vi "ArrayLast_D.vi"(11 "1D Array In":dbl[](array[numeric])) -> (0 "Last Element":dbl, 1 "Head of Array":dbl[](array[numeric]))   [LabVIEW 2009]
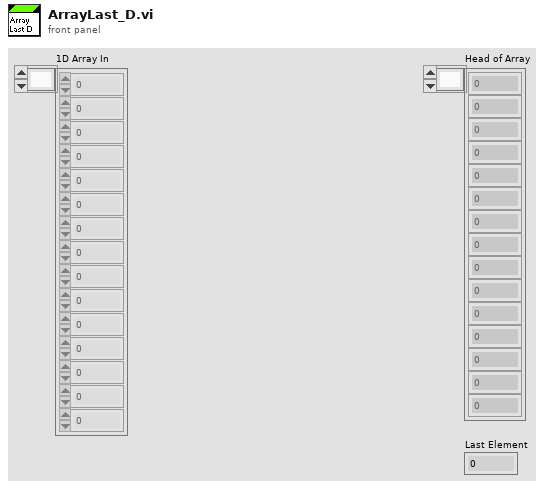
[diagram p1: front panel]
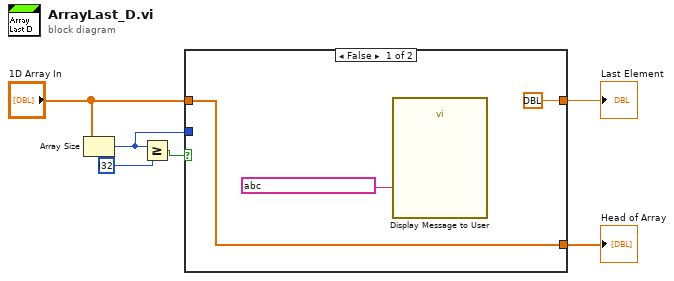
[diagram p0: block diagram]
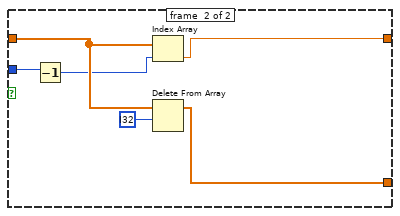
[diagram p2: hidden frame]
diagram:
  n1 = Array Size(array="1D Array In") -> (size(s)=w1:i32)
  n2 = Greater Or Equal?(x=w1, y=i32 ?) -> (x >= y?=w5:bool)
  n3 = case shown="False" w5 {
    tunnel: "1D Array In" -> [w8 w13]
    tunnel: [dbl ? ("Numeric") w15] -> w3
    tunnel: [w8 w12] -> w2
    tunnel: w1 -> [_ w11]
    frame #0 {
      n4 = call "Display Message to User"("Message"=string ?) -> ()  [unwired: 9 in, 2 out]
    }
    frame #1 {
      n5 = Decrement(x=w11) -> (x-1=w10:i32)
      n6 = Index Array(array=w13, index=w10) -> (element=w15:dbl)
      n7 = Delete From Array(array=w13, length=i32 ?) -> (array with subset deleted=w12:dbl[])  [unwired: 1 in, 1 out]
    }
  }
  "Last Element" <- w3
  "Head of Array" <- w2
